vi "Update Splash.vi"(8 "error in (no error)":errorcluster, 10 "Status":string, 11 "Plugin Splash in":refnum<class "Plugin Splash.lvclass">) -> (0 "error out":errorcluster, 3 "Plugin Splash out":refnum<class "Plugin Splash.lvclass">)   [LabVIEW 2020, in "Volatus.lvlib" / "Plugin Splash.lvclass"]
uses:
  Plugin Splash.lvclass
  Plugin Splash.lvclass/Plugin Splash.ctl
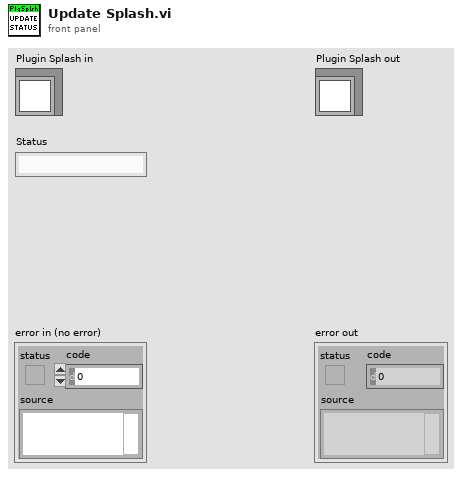
[diagram p1: front panel]
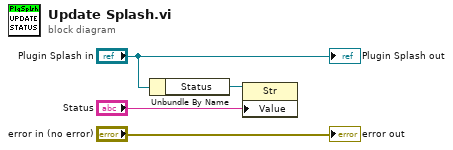
[diagram p0: block diagram]
diagram:
  n1 = Unbundle By Name("Plugin Splash in") -> ("Status"=w2:refnum<vi>)
  n2 = property class="Str"(reference=w2, "Value"="Status") -> ()  [unwired: 1 in, 2 out]
  "error out" <- "error in (no error)"
  "Plugin Splash out" <- "Plugin Splash in"
